vi "encodeStream.vi"(8 "error in (no error)":errorcluster, 11 "tBSONBinary in":refnum<class "tBSONBinary.lvclass">) -> (0 "error out":errorcluster, 2 "Byte Array":u8[](array[numeric]), 3 "tBSONBinary out":refnum<class "tBSONBinary.lvclass">)   [LabVIEW 2013, in "BSON.lvlib" / "tBSONBinary.lvclass"]
uses:
  tBSONBinary.lvclass
  tBSONElement/tBSONElement.lvclass
  getSubtype.vi
  getValue.vi
  BSON.lvlib
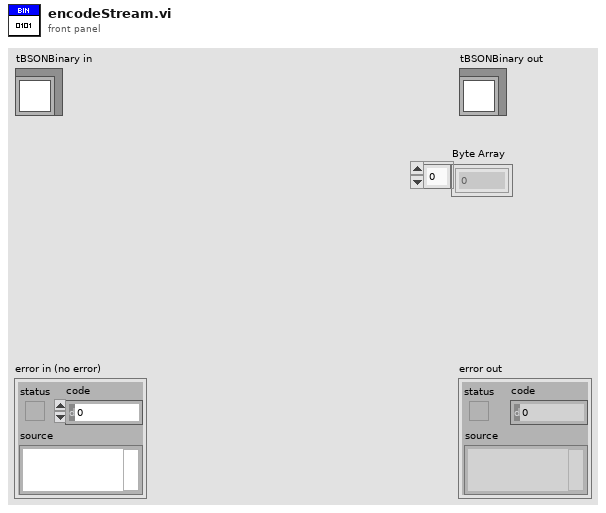
[diagram p1: front panel]
types:
  T1 = typedef "BSON.lvlib/tBSONBinary.lvclass/Subtype.ctl" = u8
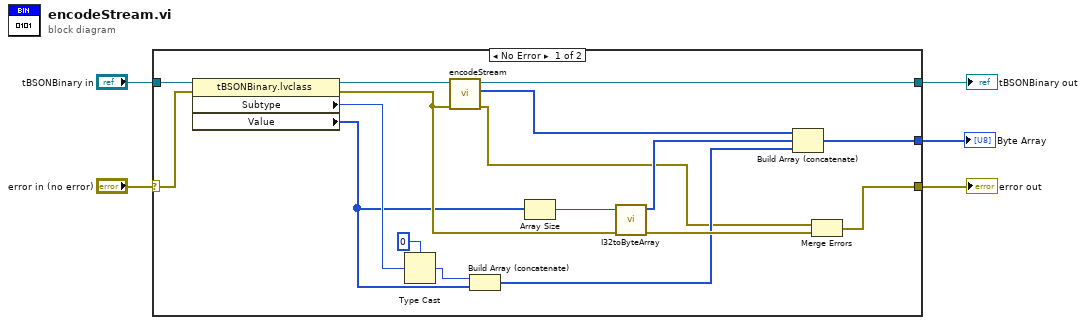
[diagram p0: block diagram]
diagram:
  n1 = case shown="No Error" "error in (no error)" {
    selector: "error in (no error)" -> [w21 w23]
    tunnel: "tBSONBinary in" -> [w22 w24]
    tunnel: [w8 w24] -> w4
    tunnel: [w19 w23] -> w2
    tunnel: [w20 _] -> w3
    frame No Error {
      n2 = property class="tBSONBinary.lvclass"(reference=w22, error in=w21) -> (reference out=w12:refnum<class "tBSONBinary.lvclass">, error out=w11:errorcluster, "Subtype"=w17:T1, "Value"=w7:u8[])
      n3 = Type Cast(type=u8 0, x=w17) -> (*(type *) &x=w16:u8)
      n4 = call-parent "encodeStream.vi"("error in (no error)"=w11, "tBSONElement in"=w12) -> ("error out"=w10:errorcluster, "Byte Array"=w9:u8[], "tBSONElement out"=w8:refnum<class "tBSONBinary.lvclass">)  [unwired: 7 in]
      n5 = Build Array (concatenate)(w16, w7) -> (w13:u8[])
      n6 = Array Size(array=w7) -> (size(s)=w6:i32)
      n7 = call "I32toByteArray.vi"("error in (no error)"=w11, "I32"=w6) -> ("error out"=w14:errorcluster, "LittleEndianByteArray"=w15:u8[])  [unwired: 8 in]
      n8 = Build Array (concatenate)(w9, w15, w13) -> (w20:u8[])
      n9 = Merge Errors(w10, w14) -> (w19:errorcluster)
    }
    frame Error {
    }
  }
  "error out" <- w2
  "tBSONBinary out" <- w4
  "Byte Array" <- w3
